vi "TERMOMETRO.vi"() -> ()   [LabVIEW 2020]
panel:
  out "?":dbl
  out "?":dbl
  in  "Thermometer 2":dbl(slide) scale=0.0..100.0
  out "Meter":dbl(knob) scale=0.0..100.0
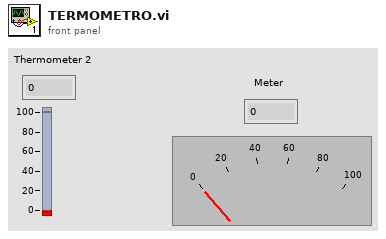
[diagram p1: front panel]
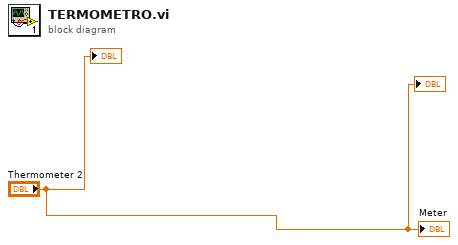
[diagram p0: block diagram]
diagram:
  "Meter" <- "Thermometer 2"
  "?" <- "Thermometer 2"
  "?" <- "Thermometer 2"
